vi "Write Name.vi"(8 "error in":errorcluster, 10 "Name":string, 11 "Engine in":refnum<class "Engine Parent Editor Node.lvclass">) -> (0 "error out":errorcluster, 3 "Engine out":refnum<class "Engine Parent Editor Node.lvclass">)   [LabVIEW 2013, in "PL Framework Configuration Tool.lvlib" / "Engine Parent Editor Node.lvclass"]
uses:
  Engine Parent Editor Node.lvclass
  <vilib>/NI/CEF/CEF_TreeControl/serializable configuration/set metadata property.vi
  TBM Configuration Node/TBM Configuration Node.lvclass
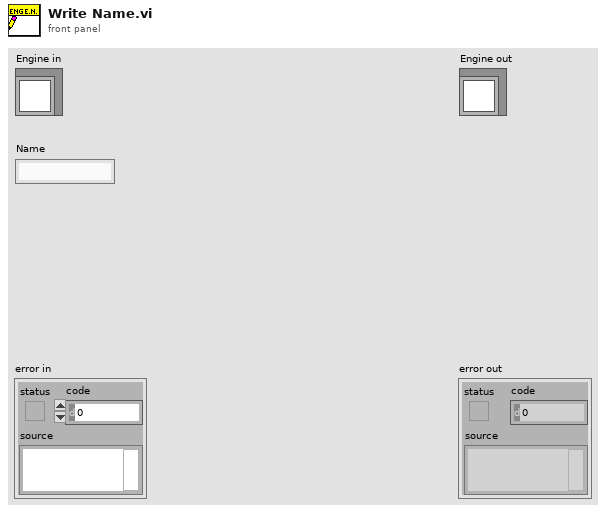
[diagram p1: front panel]
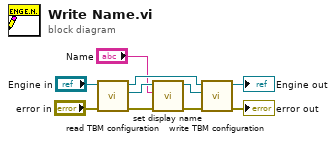
[diagram p0: block diagram]
diagram:
  n1 = call-dynamic "read TBM configuration.vi"("error in"="error in", "TBM Configuration Node in"="Engine in") -> ("error out"=w5:errorcluster, "configuration"=w4:refnum<class "TBM configuration.lvclass">, "TBM Configuration Node out"=w10:refnum<class "Engine Parent Editor Node.lvclass">)  [unwired: 7 in]
  n2 = call "set display name.vi"("error in"=w5, "display name"="Name", "configuration in"=w4) -> ("error out"=w2:errorcluster, "configuration out"=w3:refnum<class "TBM configuration.lvclass">)  [unwired: 7 in]
  n3 = call-dynamic "write TBM configuration.vi"("error in"=w2, "configuration"=w3, "TBM Configuration Node in"=w10) -> ("error out"=→"error out":errorcluster, "TBM Configuration Node out"=→"Engine out":refnum<class "Engine Parent Editor Node.lvclass">)  [unwired: 7 in]
